vi "5.3-Rotate Lidar Data.vi"(2 "Y":dbl, 3 "X":dbl, 4 "Heading (Degrees)":dbl) -> (0 "Y'":dbl, 1 "X'":dbl)   [LabVIEW 2010]
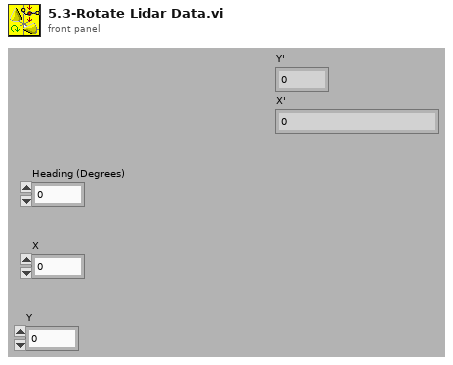
[diagram p1: front panel]
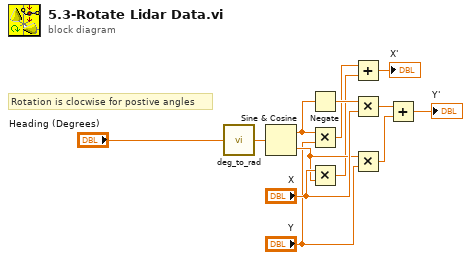
[diagram p0: block diagram]
diagram:
  # "Rotation is clocwise for postive angles"
  n1 = call "deg_to_rad.vi"("Degrees"="Heading (Degrees)") -> ("Radians"=w12:dbl)
  n2 = Sine & Cosine(0:w12) -> (1:w10:dbl, 2:w8:dbl)
  n3 = Negate(x=w10) -> (-x=w11:dbl)
  n4 = Multiply(x=w10, y="Y") -> (x*y=w3:dbl)
  n5 = Multiply(x="X", y=w8) -> (x*y=w2:dbl)
  n6 = Add(x=w3, y=w2) -> (x+y=→"X'":dbl)
  n7 = Multiply(x=w11, y="X") -> (x*y=w5:dbl)
  n8 = Multiply(x=w8, y="Y") -> (x*y=w6:dbl)
  n9 = Add(x=w5, y=w6) -> (x+y=→"Y'":dbl)
